vi "FGV-GlobalEventQueues(lvlibp).vi"(6 "Create? (F)":bool, 8 "error in (no error)":errorcluster) -> (0 "error out":errorcluster, 2 "CreatedQueue":refnum<queue>, 3 "Queue":refnum<queue>[](array[refnum]))   [LabVIEW 2017, in "Communicable State Machine.lvlib"]
uses:
  Communicable State Machine.lvlib
  Typedef/_CSM_GlobalLog_MSG.ctl
  Typedef/_CSM_Response Source Message.ctl
  Typedef/_CSM_GlobalLog_MSG_TYPE.ctl
  FGV-GlobalEventQueues.vi
  _Shared/CSM Shared.lvlib
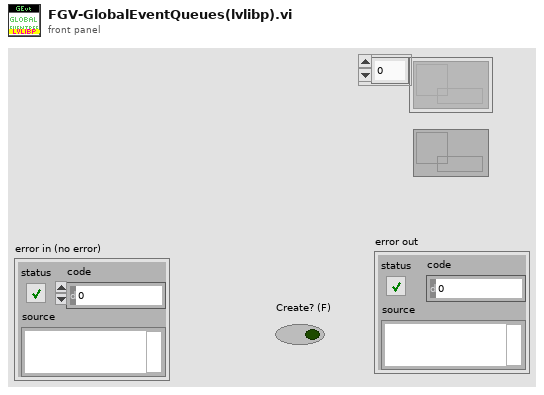
[diagram p1: front panel]
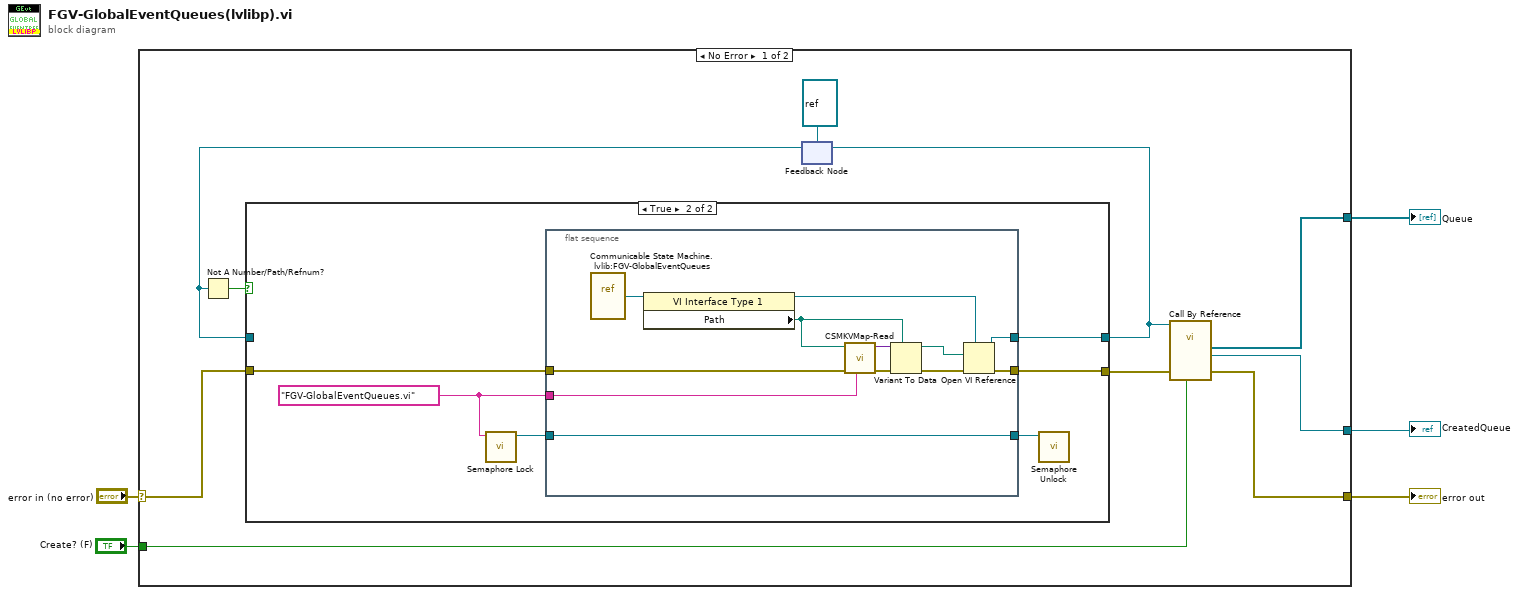
[diagram p0: block diagram]
diagram:
  n1 = case shown="No Error" "error in (no error)" {
    selector: "error in (no error)" -> [w11 w36]
    tunnel: [w8 _] -> w5
    tunnel: [w10 w36] -> w3
    tunnel: "Create? (F)" -> [w6 _]
    tunnel: [w7 _] -> w1
    frame No Error {
      n2 = feedback #1(refnum<vi> refnum) -> (w14:refnum<vi>)
      n3 = Not A Number/Path/Refnum?(number/path/refnum=w14) -> (NaN/Path/Refnum?=w15:bool)
      n4 = case shown="True" w15 {
        tunnel: [w16 w22] -> w13
        tunnel: [w17 w23] -> w12
        tunnel: w11 -> [w17 w21]
        tunnel: w14 -> [w16 _]
        frame False {
        }
        frame True {
          w20 = "FGV-GlobalEventQueues.vi" ("name")
          n5 = call "Semaphore Lock.vi"("name"=w20) -> ("semaphore"=w18:refnum<queue>)  [unwired: 10 in]
          n6 = flat-sequence {
            tunnel: [w31] -> w23
            tunnel: [w29] -> w22
            tunnel: w21 -> [w27]
            tunnel: w20 -> [w25]
            tunnel: [w24] -> w19
            tunnel: w18 -> [w24]
            frame #0 {
              n7 = vi-ref "Communicable State Machine.lvlib:FGV-GlobalEventQueues.vi"() -> (w26:refnum<vi>)
              n8 = property class="VI Interface Type 1"(reference=w26) -> (reference out=w28:refnum<vi>, "Path"=w30:path)  [unwired: 1 in, 1 out]
              n9 = call "CSMKVMap-Read.vi"("name"=w25, "Error in"=w27, "default value (empty variant)"=w30) -> ("Error out"=w35:errorcluster, "value"=w34:variant)  [unwired: 5 in]
              n10 = Variant To Data(error in=w35, type=w30, Variant=w34) -> (data=w33:path, error out=w32:errorcluster)
              n11 = Open VI Reference(type specifier VI Refnum (for type only)=w28, vi path=w33, error in (no error)=w32) -> (vi reference=w29:refnum<vi>, error out=w31:errorcluster)  [unwired: 3 in]
            }
          }
          n12 = call "Semaphore Unlock.vi"("semaphore"=w19) -> ()  [unwired: 11 in]
        }
      }
      n13 = feedback-in #1(w13) -> ()
      n14 = call-by-ref "?"(reference=w13, "Create? (F)"=w6, "error in (no error)"=w12) -> ("error out"=w10:errorcluster, "CreatedQueue"=w7:refnum<queue>, "Queue"=w8:refnum<queue>[])  [unwired: 8 in, 2 out]
    }
    frame Error {
    }
  }
  "Queue" <- w5
  "error out" <- w3
  "CreatedQueue" <- w1
